vi "Read Config Unitest.vi"(8 "error in (no error)":errorcluster, 11 "main ref":T1) -> (0 "error out":errorcluster)   [LabVIEW 2025]
uses:
  controls/LAB-IQ UI Data.ctl
  Config file  FGV Unitest enum.ctl
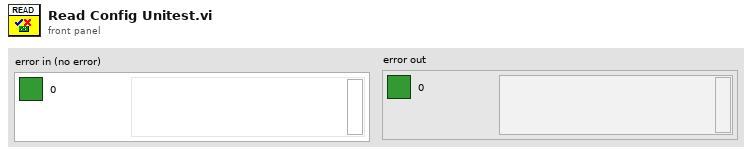
[diagram p1: front panel]
types:
  T1 = typedef "LAB-IQ UI Data.ctl" = cluster{"Main Home Screen":cluster{"GUI":refnum<vi>, "Platform Settings":refnum<vi>, "Configure":refnum<vi>, "Home":refnum<vi>, "EXIT":refnum<vi>, "service 2":refnum<vi>, "MainPage":refnum<vi>, "Analysis":refnum<vi>}, "Platform Settings":cluster{"mm/s  Surge":refnum<vi>, "Update Surge Speed":refnum<vi>, "Drive Error":refnum<vi>, "Disable Axis Jog Soft Limits":refnum<vi>, "mm/s  Sway":refnum<vi>, "Sway and Surge COM Status":refnum<vi>, "Heave COM Status":refnum<vi>, "Enable Platform":refnum<vi>, "Surge Forward Main":refnum<vi>, "Sway Right Main":refnum<vi>, "Sway Left Main":refnum<vi>, "Heave Down Main":refnum<vi>, "Heave Up main":refnum<vi>, "Update Sway Speed":refnum<vi>, "Update Heave Speed":refnum<vi>, "mm/s Heave":refnum<vi>, "mm/sec":refnum<vi>, "mm":refnum<vi>, "Surge Backward Main":refnum<vi>}, "Analysis Screen":cluster{"Analysis Home":refnum<vi>, "Surface Analysis":refnum<vi>, "Imaging":refnum<vi>, "Image Analysis":refnum<vi>, "Post Analysis":refnum<vi>}, "Config Screen":cluster{"Select Load Head":refnum<vi>, "Notes :":refnum<vi>, "FILE":refnum<vi>, "Sample ID :":refnum<vi>, "Operator ID :":refnum<vi>, "Operator Name :":refnum<vi>, "Auto":refnum<vi>}, "Motion Module":cluster{"zNL":refnum<vi>, "NL disp":refnum<vi>, "Rotary Tab":refnum<vi>, "Motion Direction:  3":refnum<vi>, "E.Velocity 2":refnum<vi>, "e.v/ssr 2":refnum<vi>, "Enter Fixed E.Velocity 2":refnum<vi>, "Enter Final SRR 2":refnum<vi>, "Enter initial SRR 2":refnum<vi>, "Enter Fixed SRR 2":refnum<vi>, "Enter the Final E.Velocity (m/s) 2":refnum<vi>, "Enter initial E.Velocity (m/s) 2":refnum<vi>, "Final Speed (RPM) 3":refnum<vi>, "Initial Speed (RPM) 2":refnum<vi>, "Enter the Final Velocity (m/s) 3":refnum<vi>, "Enter initial Velocity (m/s)  3":refnum<vi>, "Ramp Up 2":refnum<vi>, "TEST SELECTION":refnum<vi>, "SPEED SELECTION : ":refnum<vi>, "Angular Oscillation Set":refnum<vi>, "Traction":refnum<vi>, "Step Speed":refnum<vi>, "StepTable For Load-Speed":refnum<vi>, "StepTable For Speed":refnum<vi>, "Surge Forward MM":refnum<vi>, "Surge Backward MM":refnum<vi>, "M3 Image":refnum<vi>, "String 39":refnum<vi>, "Sway Left MM":refnum<vi>, "Sway Right MM":refnum<vi>, "Disable Axis Jog Soft Limits":refnum<vi>, "mm":refnum<vi>, "Heave Down MM":refnum<vi>, "Heave Up MM":refnum<vi>, "Wear Track Diameter (mm)":refnum<vi>, "Set WTD":refnum<vi>, "HomeScratch":refnum<vi>, "HomeRot":refnum<vi>, "PlaceModule":refnum<vi>, "Enter the Angle (Deg)":refnum<vi>, "Enter the Frequency (Hz)":refnum<vi>, "Motion Mode:":refnum<vi>, "LR Sway":refnum<vi>, "Rot Hor":refnum<vi>, "Scratch":refnum<vi>, "LR Cam":refnum<vi>, "MMBack":refnum<vi>, "MMNext":refnum<vi>, "Rot Ver":refnum<vi>, "Rotary Module Selection":refnum<vi>, "calculate rotary":refnum<vi>, "SPEED SELECTION : rotary":refnum<vi>, "Import 2":refnum<vi>, "Save 2":refnum<vi>, "File Path :  2":refnum<vi>, "String 45":refnum<vi>, "StepTable For Speed 3":refnum<vi>, "Enter the Speed(mm/sec)":refnum<vi>, "Enter the Speed(RPM)":refnum<vi>, "Enter Scratch Speed (mm/s):":refnum<vi>, "SwaySpeed Set":refnum<vi>, "Scartch Offset":refnum<vi>, "Motion type:":refnum<vi>, "HomeScratch 2":refnum<vi>, "Enter Scratch length (mm):":refnum<vi>, "Wear Track Diameter":refnum<vi>, "Rotary Speed Exced":refnum<vi>, "Scratch Mode":refnum<vi>, "No of Scratch":refnum<vi>}, "Environmental control":cluster{"Humidity  Status  3":refnum<vi>, "Low Temp  Status  2":refnum<vi>, "TK4 status 2":refnum<vi>, "Stage Temperature":refnum<vi>, "Sample Temperature":refnum<vi>, "Humidity (Amb)":refnum<vi>, "Clear List":refnum<vi>, "Add to list":refnum<vi>, "Wear":refnum<vi>, "Vibration":refnum<vi>, "Humidity (Chamber)":refnum<vi>, "Temperature (Chamber)":refnum<vi>, "ECR ":refnum<vi>, "Temperature (Amb)":refnum<vi>, "Microphone":refnum<vi>, "Acoustic Emission 3":refnum<vi>, "SNext":refnum<vi>, "APBack":refnum<vi>, "Enter the Temperature (°C):":refnum<vi>, "Enter the Stage \nTemperature (°C):":refnum<vi>, "Enter the Humidity (%Rh):":refnum<vi>, "Low Temp":refnum<vi>, "High Temp":refnum<vi>, "Humidity":refnum<vi>, "Sensors Picked":refnum<vi>}, "About Screen":cluster{"Password":refnum<vi>, "Home Service":refnum<vi>, "Advanced Setting":refnum<vi>, "About Tab":refnum<vi>, "ECR Port:":refnum<vi>, "Ramp Port:":refnum<vi>, "Installation/Replacement completed":refnum<vi>, "Loahead":refnum<vi>, "Heave and Surge COM Port:":refnum<vi>, "Sway COM Port:":refnum<vi>, "Temp Modbus:":refnum<vi>, "Humidity Port:":refnum<vi>, "Edit Gain Constants":refnum<vi>, "Save Gain Constants":refnum<vi>}, "Main Screen":cluster{"Main Screen Tab":refnum<vi>, "Angle and Frequency":refnum<vi>, "Stroke (mm)":refnum<vi>, "Angle (Deg)":refnum<vi>, "Main Speed Tab":refnum<vi>, "MTM MOTOR DISPLAY":refnum<vi>, "Disc Speed (m/sec)":refnum<vi>, "Ball Speed (m/sec)":refnum<vi>, "Disc Speed (RPM)":refnum<vi>, "Ball Speed (RPM)":refnum<vi>, "SPEED TAB":refnum<vi>, "Speed (m/sec)":refnum<vi>, "Set Speed (m/sec)":refnum<vi>, "Speed (RPM)":refnum<vi>, "Set Speed":refnum<vi>, "Time Tab":refnum<vi>, "Time ( HH:MM:SS ) 2":refnum<vi>, "Test Duration":refnum<vi>, "Test Duration 4":refnum<vi>, "TEST CYCLE":refnum<vi>, "TOTAL CYCLES":refnum<vi>, "Set Load (N)":refnum<vi>, "Temp Tabs":refnum<vi>, "Heater":refnum<vi>, "TK4 status":refnum<vi>, "ChamberTemp":refnum<vi>, "SetTmp":refnum<vi>, "Controller  Status":refnum<vi>, "ChamberTemp 2":refnum<vi>, "SetTmp 2":refnum<vi>, "Controller  Status 2":refnum<vi>, "ChamberTemp 3":refnum<vi>, "SetTmp 3":refnum<vi>, "Cooling":refnum<vi>, "Load Communication":refnum<vi>, "Ambient \nTemperature":refnum<vi>, "HumCOMStatus":refnum<vi>, "Ambient\n Humidity":refnum<vi>, "Freq (Hz)":refnum<vi>, "Load En":refnum<vi>, "NLt":refnum<vi>, "zNL 2":refnum<vi>, "Humidity On":refnum<vi>, "humidity disp":refnum<vi>, "Set Humidity":refnum<vi>, "NL disp 2":refnum<vi>, "Humidity On 2":refnum<vi>, "humidity disp 2":refnum<vi>, "Set Humidity 2":refnum<vi>, "NL disp 3":refnum<vi>, "AppLoadSeq scratch":refnum<vi>, "Stop Scratch":refnum<vi>, "ClrLog":refnum<vi>, "Trip Log":refnum<vi>, "STOP":refnum<vi>, "Start Test":refnum<vi>, "Test status":refnum<vi>, "AR Led":refnum<vi>, "Data":refnum<vi>, "Health":refnum<vi>, "Sway COM Status":refnum<vi>, "Heave COM Status":refnum<vi>, "Grp Tab":refnum<vi>, "Sub Graph":refnum<vi>, "SD (mm)":refnum<vi>, "Siliding distance Reset Graph":refnum<vi>, "SDGp":refnum<vi>, "Humidity Reset Graph":refnum<vi>, "HumrGp":refnum<vi>, "Acoustic Emission (mV)":refnum<vi>, "Aqucostic Reset Graph":refnum<vi>, "gACQUOS":refnum<vi>, "ECR RESET":refnum<vi>, "ECR":refnum<vi>, "Temperature Reset":refnum<vi>, "Acoustic Emission (mV) 2":refnum<vi>, "Aqucostic Reset Graph 2":refnum<vi>, "gACQUOS 2":refnum<vi>, "ECR RESET 2":refnum<vi>, "ECR 2":refnum<vi>, "Temperature Reset 2":refnum<vi>, "Temperature (deg c)":refnum<vi>, "Speed Reset Graph":refnum<vi>, "Speed Tab":refnum<vi>, "MTM DISC  SPEED":refnum<vi>, "MTM BALL SPEED":refnum<vi>, "speed mm/sec":refnum<vi>, "Hymidity":refnum<vi>, "Humidity Disable trip":refnum<vi>, "CoF Trip  2":refnum<vi>, "Depth Trip":refnum<vi>, "Weart Deapth":refnum<vi>, "Depth Reset Graph":refnum<vi>, "Weart":refnum<vi>, "Depthz":refnum<vi>, "Depth (µm)":refnum<vi>, "WearGp":refnum<vi>, "NL Trip 2":refnum<vi>, "Load pid":refnum<vi>, "Load Disable Trip":refnum<vi>, "Load Reset Graph":refnum<vi>, "NL Display 4":refnum<vi>, "Main Chart 3":refnum<vi>, "BACK":refnum<vi>, "Depth Trip 2":refnum<vi>, "COF TRIP ":refnum<vi>, "Friction Force (N)":refnum<vi>, "FF Reset Graph":refnum<vi>, "FF Disable Trip":refnum<vi>, "FF TRIP":refnum<vi>, "COF Disable Trip":refnum<vi>, "COF Reset Graph":refnum<vi>, "Start Test Temp":refnum<vi>, "zFF":refnum<vi>, "Friction Force (N) Graph":refnum<vi>, "Coefficient of Friction":refnum<vi>, "Scratch Start Test":refnum<vi>, "FF Tab":refnum<vi>, "Cyclic Friction Force (N)":refnum<vi>, "CZ FF":refnum<vi>, "Cyclic Friction Force (N) Graph":refnum<vi>, "Cyclic Coefficient of Friction":refnum<vi>, "Cyclic FF TRIP":refnum<vi>, "Cyclic FF Disable Trip":refnum<vi>, "cyclic COF Disable Trip":refnum<vi>, "cyclic COF TRIP":refnum<vi>, "cyclic COF Reset Graph":refnum<vi>, "Cyclic FF Reset Graph":refnum<vi>, "Test Trip":refnum<vi>, "Multi Scratch Pass":refnum<vi>, "Scratch Start Recording":refnum<vi>}, "Loading":cluster{"Indentation":refnum<vi>, "Reference Sample":refnum<vi>, "Load Cell Communication Slide":refnum<vi>, "com 3":refnum<vi>, "com":refnum<vi>, "DecaForce COM Status":refnum<vi>, "Update":refnum<vi>, "Clear 3":refnum<vi>, "seq":refnum<vi>, "Stribeck table":refnum<vi>, "Stribeck Table  For loading":refnum<vi>, "Loading Mode":refnum<vi>, "Enter the Final Load (N)":refnum<vi>, "Enter the CoF Trip":refnum<vi>, "Enter the Friction Force Trip":refnum<vi>, "Enter the Normal load Trip":refnum<vi>, "Enter the Load  (N)":refnum<vi>, "KiloForce":refnum<vi>, "DecaForce ":refnum<vi>, "MicroForce":refnum<vi>, "LHBack":refnum<vi>, "LHNext":refnum<vi>, "Enter the Loading Rate (N/min)":refnum<vi>, "Message":refnum<vi>, "Warning 2":refnum<vi>, "SSP 0.75":refnum<vi>, "SSP 0.5":refnum<vi>, "SSP 0.3":refnum<vi>, "Warning":refnum<vi>, "gui GIF":refnum<vi>, "Communication is established":refnum<vi>, "AppLoad 4":refnum<vi>, "Multipoint":refnum<vi>, "Load Selection":refnum<vi>}, "PID":cluster{"Ramp MulFac":refnum<vi>, "pulses LoadDiffRamp(2..10)":refnum<vi>, "PulseControlRamp(diff<=3N)":refnum<vi>, "SetLoadDeadband(%) Load(0-10N)":refnum<vi>, "PID gains out delay (microForce)":refnum<vi>, "Ramp":refnum<vi>, "Gain 2":refnum<vi>, "pulses LoadDiff(2..10)":refnum<vi>, "pulses LoadDiff(11..50)":refnum<vi>, "PulseControl(diff<=3N)":refnum<vi>, "SetLoadDeadband(%)  2":refnum<vi>, "Dummy Run":refnum<vi>, "Vertical load (N)":refnum<vi>, "AutoTune":refnum<vi>, "Offset 3 ":refnum<vi>, "apply load":refnum<vi>, "Offset  3":refnum<vi>, "apply load 2":refnum<vi>, "Enter ByPass Load":refnum<vi>, "reinit 3":refnum<vi>, "output range delay":refnum<vi>, "PID gains out delay":refnum<vi>, "Bypass Load":refnum<vi>, "pulsesSent":refnum<vi>, "pulses ":refnum<vi>, "actpid":refnum<vi>, "gFF Rot":refnum<vi>, "pulses LoadDiff(21..1000)":refnum<vi>, "Delay":refnum<vi>, "deadband":refnum<vi>}, "Config Parameters":cluster{"Tab Control 3":refnum<vi>, "Tab Control 19":refnum<vi>, "SAMPLES":refnum<vi>, "Re-initilaize":refnum<vi>, "Filter ON/OFF":refnum<vi>, "TracHomeSurgeOffsetCounts 10MM":refnum<vi>, "TracHomeSwayOffsetCounts 10MM":refnum<vi>, "Acoustic Emission:":refnum<vi>, "Apply Filter (FF)":refnum<vi>, "Filter% 2":refnum<vi>, "Apply Filter (Load)":refnum<vi>, "Filter% ":refnum<vi>, "Sway distance (mm)":refnum<vi>, "Surge distance (mm)":refnum<vi>, "DataSavingLoopDelay(ms)":refnum<vi>, "SAVE 2":refnum<vi>, "Enter Distance":refnum<vi>, "Sway Counts:":refnum<vi>, "Distance (mm): 3":refnum<vi>, "Surge Counts:":refnum<vi>, "Distance (mm): 2":refnum<vi>, "Distance (mm):":refnum<vi>, "Heave Counts:":refnum<vi>, "LRMHomeSurgeOffsetCounts":refnum<vi>, "LRMHomeSwayOffsetCounts":refnum<vi>, "TracHomeSurgeOffsetCounts 20MM":refnum<vi>, "TracHomeSwayOffsetCounts 20MM":refnum<vi>, "RotHomeSwayOffsetCounts":refnum<vi>, "RotHomeSurgeOffsetCounts":refnum<vi>, "Heave distance":refnum<vi>, "Zmm":refnum<vi>, "Heave Pulses/mm":refnum<vi>, "Surge Pulses/mm":refnum<vi>, "Sway Pulses/mm":refnum<vi>, "Heave Pitch":refnum<vi>, "Surge Pitch":refnum<vi>, "Sway Pitch":refnum<vi>, "Heave PPR":refnum<vi>, "Surge PPR":refnum<vi>, "Sway PPR":refnum<vi>, "Tab Control 5":refnum<vi>, "Tab Control 14":refnum<vi>, "Tab Control 26":refnum<vi>, "AE":refnum<vi>, "Heave Loop Delay":refnum<vi>, "Heave PID Speed":refnum<vi>, "Surge Jog Speed":refnum<vi>, "Heave Jog Speed":refnum<vi>, "Sway Loop Delay":refnum<vi>, "Sway PID Speed":refnum<vi>, "Sway Jog Speed":refnum<vi>, "DEPTH TRIP VALUE":refnum<vi>, "LOAD TRIP VALUE":refnum<vi>, "DEPTH TRIP   ENABLE":refnum<vi>, "LOAD TRIP  ENABLE":refnum<vi>, "CYCLIC FF TRIP VALUE":refnum<vi>, "FF TRIP VALUE":refnum<vi>, "CYCLIC CoF TRIP VALUE":refnum<vi>, "COF TRIP VALUE":refnum<vi>, "CYCLIC COF TRIP  ENABLE":refnum<vi>, "CYCLIC FF TRIP  ENABLE":refnum<vi>, "FF TRIP  ENABLE":refnum<vi>, "COF TRIP  ENABLE":refnum<vi>}, "Loading Com Port":cluster{"ClearAll":refnum<vi>, "Mz(Nm)":refnum<vi>, "My(Nm)":refnum<vi>, "Mx(Nm)":refnum<vi>, "Save Dwell":refnum<vi>, "Mx ":refnum<vi>, "My ":refnum<vi>, "Mz":refnum<vi>, "Fx(N)":refnum<vi>, "Fy(N)":refnum<vi>, "Fz(N)":refnum<vi>, "ZeroAll":refnum<vi>, "Acq Delay (ms)":refnum<vi>, "Burst Delay (ms)":refnum<vi>, "model":refnum<vi>, "SN":refnum<vi>, "FFx(N)":refnum<vi>, "Sensor IP":refnum<vi>, "Port":refnum<vi>, "FFy(N)":refnum<vi>, "Load(N)":refnum<vi>, "delete Handle":refnum<vi>, "Create Handle":refnum<vi>, "ft_data":refnum<vi>, "ft_range":refnum<vi>, "ft_data 2":refnum<vi>, "stop 6":refnum<vi>, "running_flag":refnum<vi>, "ft_udp_handle":refnum<vi>, "get-data-return":refnum<vi>, "get-range-return":refnum<vi>, "zero-return":refnum<vi>, "filter-return":refnum<vi>, "initial-return":refnum<vi>, "deleteHandle-result":refnum<vi>, "Load Cell Temp":refnum<vi>}, "Heave AND Surge":cluster{"SURGE POSE":refnum<vi>, "error out Read":refnum<vi>, "HEAVE POSE":refnum<vi>, "State":refnum<vi>, "Homed":refnum<vi>, "Sequence ID":refnum<vi>, "error out Write":refnum<vi>, "faultCode":refnum<vi>, "Ack ID":refnum<vi>, "SPEED":refnum<vi>, "Distance":refnum<vi>, "Mode Command":refnum<vi>, "Heave and Surge Read":refnum<vi>, "Read Heave Temp":refnum<vi>, "Spare 15":refnum<vi>, "Spare 14":refnum<vi>, "Spare 13":refnum<vi>, "Spare 12":refnum<vi>, "Spare 11":refnum<vi>, "Spare 10":refnum<vi>, "Spare 9":refnum<vi>, "Spare 8":refnum<vi>, "Spare 7":refnum<vi>, "Spare 6":refnum<vi>, "Spare 5":refnum<vi>, "Spare 4":refnum<vi>, "Spare 2":refnum<vi>, "Spare 1":refnum<vi>, "Node Id":refnum<vi>, "Spare 3":refnum<vi>, "SPARE 4":refnum<vi>, "SPARE 3":refnum<vi>, "SPARE 2":refnum<vi>, "SPARE 1":refnum<vi>, "fwMajor":refnum<vi>, "fwMinor":refnum<vi>, "Manual Write":refnum<vi>, "Heave and Surge Write":refnum<vi>}, "New PID LOGIC":cluster{"Fine Tune Zone":refnum<vi>, "PID SDelay":refnum<vi>, "Max_pos_limit":refnum<vi>, "Min_pos_limit":refnum<vi>, "i_limit":refnum<vi>, "pct_scale":refnum<vi>, "Deadband":refnum<vi>, "Kd":refnum<vi>, "Ki":refnum<vi>, "Kp":refnum<vi>, "Current Position":refnum<vi>, "Set Load":refnum<vi>, "Current Load":refnum<vi>, "Pulse delta":refnum<vi>, "Init Step":refnum<vi>, "Max Step Linit":refnum<vi>}, "SWAY ":cluster{"fwMajor":refnum<vi>, "Homed":refnum<vi>, "Rotary POSE":refnum<vi>, "State":refnum<vi>, "SWAY POSE":refnum<vi>, "Ack ID":refnum<vi>, "faultCode":refnum<vi>, "Node Id":refnum<vi>, "fwMinor":refnum<vi>, "Spare 6":refnum<vi>, "Spare 5":refnum<vi>, "Spare 4":refnum<vi>, "Spare 3":refnum<vi>, "Spare 2":refnum<vi>, "Spare 1":refnum<vi>, "Spare 7":refnum<vi>, "SPARE  5":refnum<vi>, "error out Write  SWAY ":refnum<vi>, "error out Read SWAY ":refnum<vi>, "Manual Write SWAY ":refnum<vi>, "SWAY WRITE":refnum<vi>, "SPARE  4":refnum<vi>, "SPARE  3":refnum<vi>, "SPARE 2":refnum<vi>, "SPARE 1":refnum<vi>, "Spare 15":refnum<vi>, "Spare 14":refnum<vi>, "Spare 13":refnum<vi>, "Spare 12":refnum<vi>, "Spare 11":refnum<vi>, "Spare 9":refnum<vi>, "Spare 8":refnum<vi>, "SPEED":refnum<vi>, "Distance":refnum<vi>, "Mode Command":refnum<vi>, "Sequence ID":refnum<vi>, "SWAY READ":refnum<vi>, "Spare 10":refnum<vi>, "Read SWAY Temp":refnum<vi>}, "Analysis Screen":cluster{"Analysis Home":refnum<vi>, "Refresh 2":refnum<vi>, "MEAN 4":refnum<vi>, "SD 4":refnum<vi>, "VARIANCE 4":refnum<vi>, "MEAN  3":refnum<vi>, "SD  3":refnum<vi>, "VARIANCE  3":refnum<vi>, "MEAN 2":refnum<vi>, "SD  2":refnum<vi>, "VARIANCE 2":refnum<vi>, "MEAN":refnum<vi>, "SD":refnum<vi>, "VARIANCE":refnum<vi>, "File 4 Discription":refnum<vi>, "OPEN 4":refnum<vi>, "File Name 4":refnum<vi>, "OPEN 3":refnum<vi>, "File 3 Discription":refnum<vi>, "File Name 3":refnum<vi>, "Y-AXIS":refnum<vi>, "X-AXIS":refnum<vi>, "XY Graph":refnum<vi>, "File Name 2":refnum<vi>, "File Name 1":refnum<vi>, "OPEN 2":refnum<vi>, "OPEN 1":refnum<vi>, "File 1 Discription ":refnum<vi>, "File 2 Discription":refnum<vi>, "Export":refnum<vi>, "File Format":refnum<vi>}}
  T2 = typedef "Config file  FGV Unitest enum.ctl" = enum16{"OPEN", "READ", "WRITE", "CLOSE"}
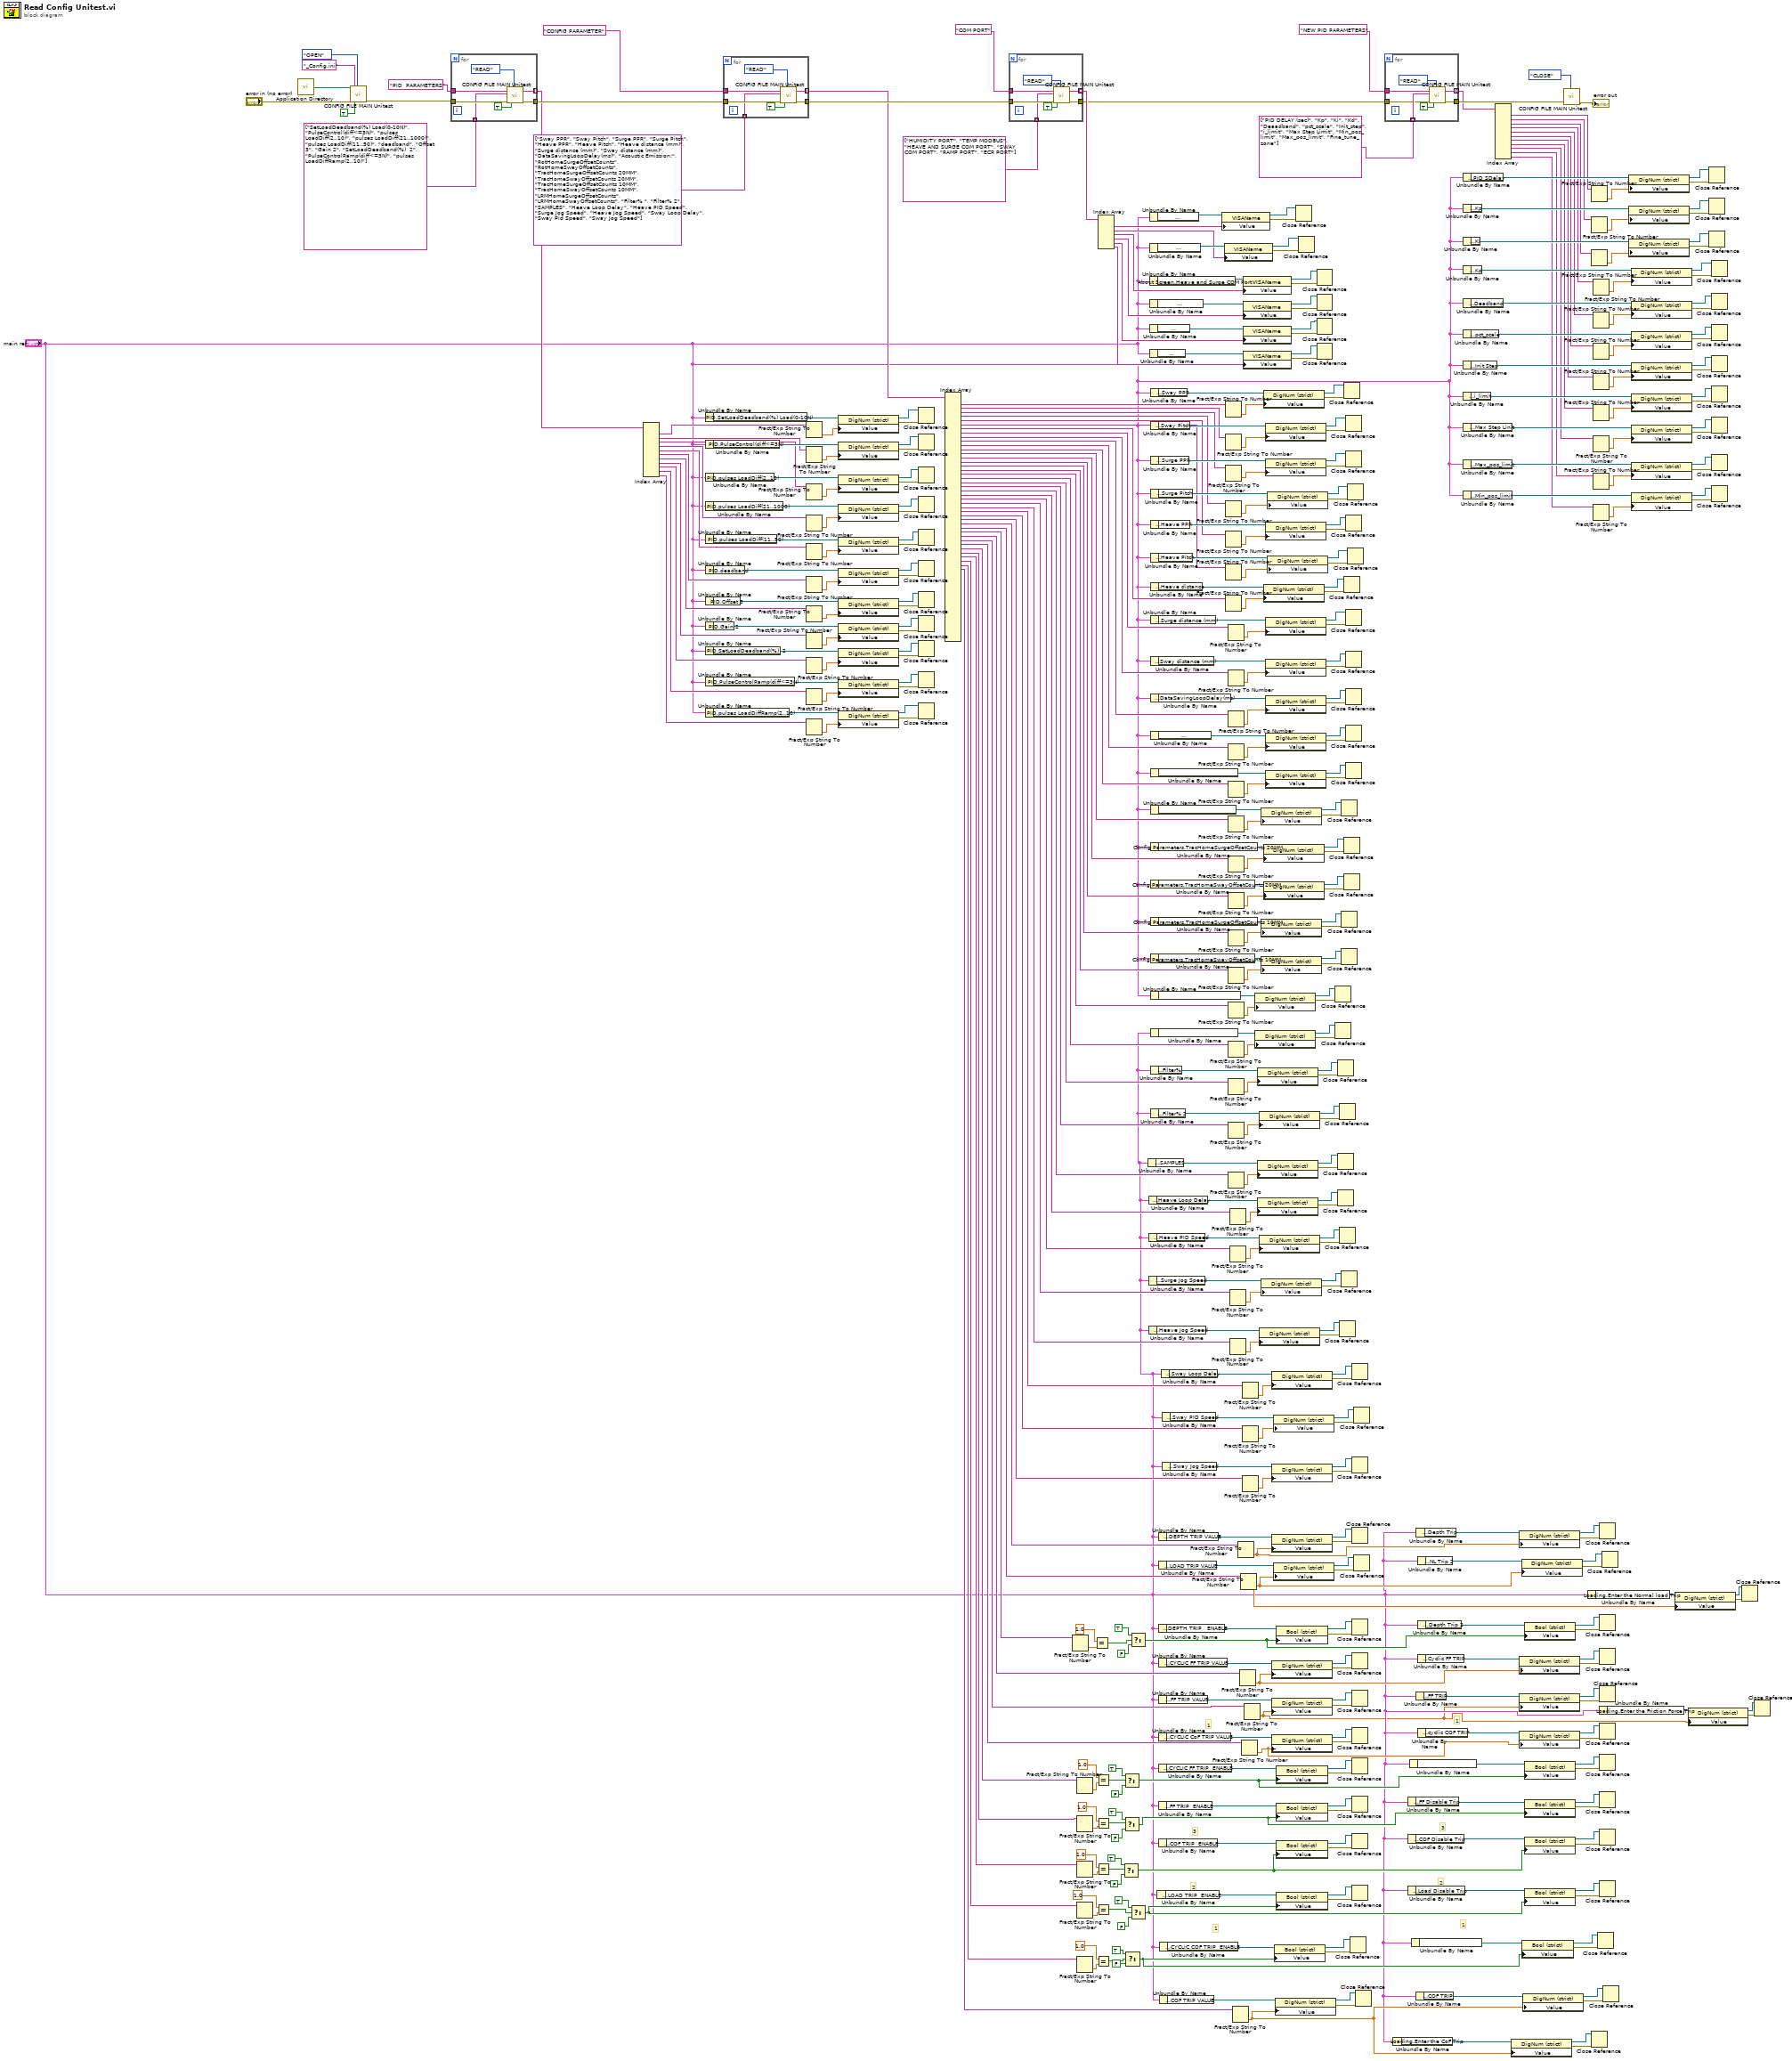
[diagram p0: block diagram]
diagram:
  # "3"
  # "2"
  # "1"
  # "1"
  # "3"
  # "2"
  # "1"
  # "1"
  n1 = call <vilib>:"Application Directory.vi"() -> ("Application Directory"=w435:path)
  n2 = call "CONFIG FILE MAIN Unitest.vi"("File Path"=w435, "error in"="error in (no error)", "file name"="_Config.ini", "PARAMETER/CONFIG"=TRUE, "Config Enum"=Config_file__FGV_Unitest_enum."OPEN") -> ("error out"=w434:errorcluster)  [unwired: 13 in, 1 out]
  n3 = for {
    tunnel: w434 -> [w446]
    tunnel: "PID  PARAMETERS" ("WRITE /READ SECTION") -> [w445]
    tunnel: string[] ["SetLoadDeadband(%) Load(0-10N)", "PulseControl(diff<=3N)", "pulses LoadDiff(2..10)", "pulses LoadDiff(21..1000)", "pulses LoadDiff(11..50)", "deadband", "Offset  3", "Gain 2", "SetLoadDeadband(%)  2", "PulseControlRamp(diff<=3N)", "pulses LoadDiffRamp(2..10)"] -> [w441] mode=indexing
    tunnel: [w444] -> w431
    tunnel: [w440] -> w244 mode=indexing
    n4 = call "CONFIG FILE MAIN Unitest.vi"("WRITE /READ SECTION"=w445, "READ KEY"=w441, "error in"=w446, "PARAMETER/CONFIG"=TRUE, "Config Enum"=Config_file__FGV_Unitest_enum."READ") -> ("READ VALUE"=w440:string, "error out"=w444:errorcluster)  [unwired: 13 in]
  }
  n5 = Index Array(array=w244) -> (element #1=w243:string, element #2=w242:string, element #3=w241:string, element #4=w240:string, element #5=w239:string, element #6=w238:string, element #7=w237:string, element #8=w236:string, element #9=w235:string, element #10=w234:string, element #11=w233:string)  [unwired: 11 in]
  n6 = Unbundle By Name("main ref") -> ("PID.SetLoadDeadband(%) Load(0-10N)"=w425:refnum<vi>)
  n7 = Unbundle By Name("main ref") -> ("PID.PulseControl(diff<=3N)"=w420:refnum<vi>)
  n8 = Unbundle By Name("main ref") -> ("PID.pulses LoadDiff(2..10)"=w419:refnum<vi>)
  n9 = Unbundle By Name("main ref") -> ("PID.pulses LoadDiff(21..1000)"=w414:refnum<vi>)
  n10 = Unbundle By Name("main ref") -> ("PID.pulses LoadDiff(11..50)"=w413:refnum<vi>)
  n11 = Unbundle By Name("main ref") -> ("PID.deadband"=w408:refnum<vi>)
  n12 = Unbundle By Name("main ref") -> ("PID.Offset 3"=w407:refnum<vi>)
  n13 = Unbundle By Name("main ref") -> ("PID.Gain 2"=w402:refnum<vi>)
  n14 = Unbundle By Name("main ref") -> ("PID.SetLoadDeadband(%)  2"=w401:refnum<vi>)
  n15 = Unbundle By Name("main ref") -> ("PID.PulseControlRamp(diff<=3N)"=w397:refnum<vi>)
  n16 = Unbundle By Name("main ref") -> ("PID.pulses LoadDiffRamp(2..10)"=w395:refnum<vi>)
  n17 = for {
    tunnel: w431 -> [w453]
    tunnel: "CONFIG PARAMETER" ("WRITE /READ SECTION") -> [w452]
    tunnel: [w451] -> w429
    tunnel: string[] ["Sway PPR", "Sway Pitch", "Surge PPR", "Surge Pitch", "Heave PPR", "Heave Pitch", "Heave distance (mm)", "Surge distance (mm)", "Sway distance (mm)", "DataSavingLoopDelay(ms)", "Acoustic Emission:", "RotHomeSurgeOffsetCounts", "RotHomeSwayOffsetCounts", "TracHomeSurgeOffsetCounts 20MM", "TracHomeSwayOffsetCounts 20MM", "TracHomeSurgeOffsetCounts 10MM", "TracHomeSwayOffsetCounts 10MM", "LRMHomeSurgeOffsetCounts", "LRMHomeSwayOffsetCounts", "Filter% ", "Filter% 2", "SAMPLES", "Heave Loop Delay", "Heave PID Speed", "Surge Jog Speed", "Heave Jog Speed", "Sway Loop Delay", "Sway Pid Speed", "Sway Jog Speed"] -> [w448] mode=indexing
    tunnel: [w447] -> w300 mode=indexing
    n18 = call "CONFIG FILE MAIN Unitest.vi"("WRITE /READ SECTION"=w452, "READ KEY"=w448, "error in"=w453, "PARAMETER/CONFIG"=TRUE, "Config Enum"=Config_file__FGV_Unitest_enum."READ") -> ("READ VALUE"=w447:string, "error out"=w451:errorcluster)  [unwired: 13 in]
  }
  n19 = Fract/Exp String To Number(string=w243) -> (number=w255:dbl)  [unwired: 3 in, 1 out]
  n20 = Fract/Exp String To Number(string=w242) -> (number=w254:dbl)  [unwired: 3 in, 1 out]
  n21 = Fract/Exp String To Number(string=w241) -> (number=w253:dbl)  [unwired: 3 in, 1 out]
  n22 = Fract/Exp String To Number(string=w240) -> (number=w252:dbl)  [unwired: 3 in, 1 out]
  n23 = Fract/Exp String To Number(string=w239) -> (number=w251:dbl)  [unwired: 3 in, 1 out]
  n24 = Fract/Exp String To Number(string=w238) -> (number=w250:dbl)  [unwired: 3 in, 1 out]
  n25 = Fract/Exp String To Number(string=w237) -> (number=w249:dbl)  [unwired: 3 in, 1 out]
  n26 = Fract/Exp String To Number(string=w236) -> (number=w248:dbl)  [unwired: 3 in, 1 out]
  n27 = Fract/Exp String To Number(string=w235) -> (number=w247:dbl)  [unwired: 3 in, 1 out]
  n28 = Fract/Exp String To Number(string=w234) -> (number=w246:dbl)  [unwired: 3 in, 1 out]
  n29 = Fract/Exp String To Number(string=w233) -> (number=w245:dbl)  [unwired: 3 in, 1 out]
  n30 = property class="DigNum (strict)"(reference=w425, "Value"=w255) -> (reference out=w423:refnum<vi>, error out=w424:errorcluster)  [unwired: 1 in]
  n31 = property class="DigNum (strict)"(reference=w420, "Value"=w254) -> (reference out=w422:refnum<vi>, error out=w421:errorcluster)  [unwired: 1 in]
  n32 = property class="DigNum (strict)"(reference=w419, "Value"=w253) -> (reference out=w417:refnum<vi>, error out=w418:errorcluster)  [unwired: 1 in]
  n33 = property class="DigNum (strict)"(reference=w414, "Value"=w252) -> (reference out=w416:refnum<vi>, error out=w415:errorcluster)  [unwired: 1 in]
  n34 = property class="DigNum (strict)"(reference=w413, "Value"=w251) -> (reference out=w411:refnum<vi>, error out=w412:errorcluster)  [unwired: 1 in]
  n35 = property class="DigNum (strict)"(reference=w408, "Value"=w250) -> (reference out=w410:refnum<vi>, error out=w409:errorcluster)  [unwired: 1 in]
  n36 = property class="DigNum (strict)"(reference=w407, "Value"=w249) -> (reference out=w405:refnum<vi>, error out=w406:errorcluster)  [unwired: 1 in]
  n37 = property class="DigNum (strict)"(reference=w402, "Value"=w248) -> (reference out=w404:refnum<vi>, error out=w403:errorcluster)  [unwired: 1 in]
  n38 = property class="DigNum (strict)"(reference=w401, "Value"=w247) -> (reference out=w399:refnum<vi>, error out=w400:errorcluster)  [unwired: 1 in]
  n39 = property class="DigNum (strict)"(reference=w397, "Value"=w246) -> (reference out=w396:refnum<vi>, error out=w398:errorcluster)  [unwired: 1 in]
  n40 = property class="DigNum (strict)"(reference=w395, "Value"=w245) -> (reference out=w393:refnum<vi>, error out=w394:errorcluster)  [unwired: 1 in]
  n41 = Close Reference(reference=w423, error in (no error)=w424) -> ()  [unwired: 1 out]
  n42 = Close Reference(reference=w422, error in (no error)=w421) -> ()  [unwired: 1 out]
  n43 = Close Reference(reference=w417, error in (no error)=w418) -> ()  [unwired: 1 out]
  n44 = Close Reference(reference=w416, error in (no error)=w415) -> ()  [unwired: 1 out]
  n45 = Close Reference(reference=w411, error in (no error)=w412) -> ()  [unwired: 1 out]
  n46 = Close Reference(reference=w410, error in (no error)=w409) -> ()  [unwired: 1 out]
  n47 = Close Reference(reference=w405, error in (no error)=w406) -> ()  [unwired: 1 out]
  n48 = Close Reference(reference=w404, error in (no error)=w403) -> ()  [unwired: 1 out]
  n49 = Close Reference(reference=w399, error in (no error)=w400) -> ()  [unwired: 1 out]
  n50 = Close Reference(reference=w396, error in (no error)=w398) -> ()  [unwired: 1 out]
  n51 = Close Reference(reference=w393, error in (no error)=w394) -> ()  [unwired: 1 out]
  n52 = Index Array(array=w300) -> (element #1=w299:string, element #2=w298:string, element #3=w297:string, element #4=w296:string, element #5=w295:string, element #6=w294:string, element #7=w293:string, element #8=w292:string, element #9=w291:string, element #10=w290:string, element #11=w289:string, element #12=w288:string, element #13=w287:string, element #14=w286:string, element #15=w285:string, element #16=w284:string, element #17=w283:string, element #18=w282:string, element #19=w281:string, element #20=w280:string, element #21=w279:string, element #22=w278:string, element #23=w216:string, element #24=w215:string, element #25=w214:string, element #26=w213:string, element #27=w139:string, element #28=w138:string, element #29=w137:string, element #30=w87:string, element #31=w86:string, element #32=w85:string, element #33=w84:string, element #34=w83:string, element #35=w82:string, element #36=w81:string, element #37=w80:string, element #38=w79:string, element #39=w78:string, element #40=w77:string, element #41=w23:string)  [unwired: 58 in, 17 out]
  n53 = for {
    tunnel: w429 -> [w460]
    tunnel: "COM PORT" ("WRITE /READ SECTION") -> [w459]
    tunnel: [w458] -> w211
    tunnel: string[] ["HUMIDITY PORT", "TEMP MODBUS", "HEAVE AND SURGE COM PORT", "SWAY COM PORT", "RAMP PORT", "ECR PORT"] -> [w455] mode=indexing
    tunnel: [w454] -> w307 mode=indexing
    n54 = call "CONFIG FILE MAIN Unitest.vi"("WRITE /READ SECTION"=w459, "READ KEY"=w455, "error in"=w460, "PARAMETER/CONFIG"=TRUE, "Config Enum"=Config_file__FGV_Unitest_enum."READ") -> ("READ VALUE"=w454:string, "error out"=w458:errorcluster)  [unwired: 13 in]
  }
  n55 = Fract/Exp String To Number(string=w85) -> (number=w99:dbl)  [unwired: 3 in, 1 out]
  n56 = Fract/Exp String To Number(string=w81) -> (number=w100:dbl)  [unwired: 3 in, 1 out]
  n57 = Fract/Exp String To Number(string=w80) -> (number=w98:dbl)  [unwired: 3 in, 1 out]
  n58 = Fract/Exp String To Number(string=w79) -> (number=w97:dbl)  [unwired: 3 in, 1 out]
  n59 = Fract/Exp String To Number(string=w78) -> (number=w96:dbl)  [unwired: 3 in, 1 out]
  n60 = Fract/Exp String To Number(string=w77) -> (number=w95:dbl)  [unwired: 3 in, 1 out]
  n61 = Equal?(x=1.0, y=w99) -> (x = y?=w60:bool)
  n62 = Equal?(x=1.0, y=w100) -> (x = y?=w63:bool)
  n63 = Equal?(x=1.0, y=w98) -> (x = y?=w64:bool)
  n64 = Equal?(x=1.0, y=w97) -> (x = y?=w65:bool)
  n65 = Equal?(x=1.0, y=w96) -> (x = y?=w66:bool)
  n66 = Equal?(x=1.0, y=w95) -> (x = y?=w88:bool)
  n67 = Index Array(array=w307) -> (element #1=w306:string, element #2=w305:string, element #3=w304:string, element #4=w303:string, element #5=w302:string, element #6=w301:string)  [unwired: 6 in]
  n68 = Select(t=TRUE, s=w65, f=FALSE) -> (s? t:f=w20:bool)
  n69 = Select(t=TRUE, s=w63, f=FALSE) -> (s? t:f=w18:bool)
  n70 = Select(t=TRUE, s=w64, f=FALSE) -> (s? t:f=w19:bool)
  n71 = Select(t=TRUE, s=w88, f=FALSE) -> (s? t:f=w22:bool)
  n72 = Select(t=TRUE, s=w60, f=FALSE) -> (s? t:f=w15:bool)
  n73 = Select(t=TRUE, s=w66, f=FALSE) -> (s? t:f=w21:bool)
  n74 = Unbundle By Name("main ref") -> ("Config Parameters.SAMPLES"=w331:refnum<vi>)
  n75 = Unbundle By Name("main ref") -> ("Config Parameters.Heave Loop Delay"=w219:refnum<vi>)
  n76 = Unbundle By Name("main ref") -> ("Config Parameters.Heave PID Speed"=w220:refnum<vi>)
  n77 = Unbundle By Name("main ref") -> ("Config Parameters.Surge Jog Speed"=w224:refnum<vi>)
  n78 = Unbundle By Name("main ref") -> ("Config Parameters.Heave Jog Speed"=w225:refnum<vi>)
  n79 = Unbundle By Name("main ref") -> ("About Screen.Humidity Port:"=w325:refnum<vi>)
  n80 = Unbundle By Name("main ref") -> ("About Screen.Temp Modbus:"=w320:refnum<vi>)
  n81 = Unbundle By Name("main ref") -> ("About Screen.Heave and Surge COM Port:"=w319:refnum<vi>)
  n82 = Unbundle By Name("main ref") -> ("About Screen.Sway COM Port:"=w315:refnum<vi>)
  n83 = Unbundle By Name("main ref") -> ("About Screen.Ramp Port:"=w314:refnum<vi>)
  n84 = Unbundle By Name("main ref") -> ("About Screen.ECR Port:"=w311:refnum<vi>)
  n85 = Unbundle By Name("main ref") -> ("Config Parameters.Sway PPR"=w392:refnum<vi>)
  n86 = Unbundle By Name("main ref") -> ("Config Parameters.Sway Pitch"=w387:refnum<vi>)
  n87 = Unbundle By Name("main ref") -> ("Config Parameters.Surge PPR"=w381:refnum<vi>)
  n88 = Unbundle By Name("main ref") -> ("Config Parameters.Surge Pitch"=w386:refnum<vi>)
  n89 = Unbundle By Name("main ref") -> ("Config Parameters.Heave PPR"=w380:refnum<vi>)
  n90 = Unbundle By Name("main ref") -> ("Config Parameters.Heave Pitch"=w376:refnum<vi>)
  n91 = Unbundle By Name("main ref") -> ("Config Parameters.Heave distance"=w370:refnum<vi>)
  n92 = Unbundle By Name("main ref") -> ("Config Parameters.Surge distance (mm)"=w374:refnum<vi>)
  n93 = Unbundle By Name("main ref") -> ("Config Parameters.Sway distance (mm)"=w368:refnum<vi>)
  n94 = Unbundle By Name("main ref") -> ("Config Parameters.DataSavingLoopDelay(ms)"=w365:refnum<vi>)
  n95 = Unbundle By Name("main ref") -> ("Config Parameters.Acoustic Emission:"=w362:refnum<vi>)
  n96 = Unbundle By Name("main ref") -> ("Config Parameters.RotHomeSurgeOffsetCounts"=w359:refnum<vi>)
  n97 = Unbundle By Name("main ref") -> ("Config Parameters.RotHomeSwayOffsetCounts"=w356:refnum<vi>)
  n98 = Unbundle By Name("main ref") -> ("Config Parameters.TracHomeSurgeOffsetCounts 20MM"=w353:refnum<vi>)
  n99 = Unbundle By Name("main ref") -> ("Config Parameters.TracHomeSwayOffsetCounts 20MM"=w350:refnum<vi>)
  n100 = Unbundle By Name("main ref") -> ("Config Parameters.TracHomeSurgeOffsetCounts 10MM"=w346:refnum<vi>)
  n101 = Unbundle By Name("main ref") -> ("Config Parameters.TracHomeSwayOffsetCounts 10MM"=w349:refnum<vi>)
  n102 = Unbundle By Name("main ref") -> ("Config Parameters.LRMHomeSurgeOffsetCounts"=w340:refnum<vi>)
  n103 = Unbundle By Name("main ref") -> ("Config Parameters.LRMHomeSwayOffsetCounts"=w337:refnum<vi>)
  n104 = Unbundle By Name("main ref") -> ("Config Parameters.Filter%"=w336:refnum<vi>)
  n105 = Unbundle By Name("main ref") -> ("Config Parameters.Filter% 2"=w332:refnum<vi>)
  n106 = Unbundle By Name("main ref") -> ("Config Parameters.LOAD TRIP  ENABLE"=w109:refnum<vi>)
  n107 = Unbundle By Name("main ref") -> ("Config Parameters.DEPTH TRIP VALUE"=w110:refnum<vi>)
  n108 = Unbundle By Name("main ref") -> ("Config Parameters.LOAD TRIP VALUE"=w114:refnum<vi>)
  n109 = Unbundle By Name("main ref") -> ("Config Parameters.DEPTH TRIP   ENABLE"=w115:refnum<vi>)
  n110 = Unbundle By Name("main ref") -> ("Config Parameters.CYCLIC FF TRIP VALUE"=w121:refnum<vi>)
  n111 = Unbundle By Name("main ref") -> ("Config Parameters.FF TRIP VALUE"=w122:refnum<vi>)
  n112 = Unbundle By Name("main ref") -> ("Config Parameters.CYCLIC CoF TRIP VALUE"=w127:refnum<vi>)
  n113 = Unbundle By Name("main ref") -> ("Config Parameters.CYCLIC FF TRIP  ENABLE"=w128:refnum<vi>)
  n114 = Unbundle By Name("main ref") -> ("Config Parameters.FF TRIP  ENABLE"=w136:refnum<vi>)
  n115 = Unbundle By Name("main ref") -> ("Config Parameters.COF TRIP  ENABLE"=w131:refnum<vi>)
  n116 = Unbundle By Name("main ref") -> ("Config Parameters.CYCLIC COF TRIP  ENABLE"=w104:refnum<vi>)
  n117 = Unbundle By Name("main ref") -> ("Config Parameters.COF TRIP VALUE"=w103:refnum<vi>)
  n118 = Unbundle By Name("main ref") -> ("Config Parameters.Sway Loop Delay"=w151:refnum<vi>)
  n119 = Unbundle By Name("main ref") -> ("Config Parameters.Sway PID Speed"=w147:refnum<vi>)
  n120 = Unbundle By Name("main ref") -> ("Config Parameters.Sway Jog Speed"=w146:refnum<vi>)
  n121 = property class="VISAName"(reference=w325, "Value"=w306) -> (reference out=w323:refnum<vi>, error out=w324:errorcluster)  [unwired: 1 in]
  n122 = property class="VISAName"(reference=w320, "Value"=w305) -> (reference out=w322:refnum<vi>, error out=w321:errorcluster)  [unwired: 1 in]
  n123 = Fract/Exp String To Number(string=w299) -> (number=w277:dbl)  [unwired: 3 in, 1 out]
  n124 = Fract/Exp String To Number(string=w298) -> (number=w276:dbl)  [unwired: 3 in, 1 out]
  n125 = Fract/Exp String To Number(string=w297) -> (number=w275:dbl)  [unwired: 3 in, 1 out]
  n126 = Fract/Exp String To Number(string=w296) -> (number=w274:dbl)  [unwired: 3 in, 1 out]
  n127 = Fract/Exp String To Number(string=w295) -> (number=w273:dbl)  [unwired: 3 in, 1 out]
  n128 = Fract/Exp String To Number(string=w294) -> (number=w272:dbl)  [unwired: 3 in, 1 out]
  n129 = Fract/Exp String To Number(string=w293) -> (number=w271:dbl)  [unwired: 3 in, 1 out]
  n130 = Fract/Exp String To Number(string=w292) -> (number=w270:dbl)  [unwired: 3 in, 1 out]
  n131 = Fract/Exp String To Number(string=w291) -> (number=w269:dbl)  [unwired: 3 in, 1 out]
  n132 = Fract/Exp String To Number(string=w290) -> (number=w268:dbl)  [unwired: 3 in, 1 out]
  n133 = Fract/Exp String To Number(string=w289) -> (number=w267:dbl)  [unwired: 3 in, 1 out]
  n134 = Fract/Exp String To Number(string=w288) -> (number=w266:dbl)  [unwired: 3 in, 1 out]
  n135 = Fract/Exp String To Number(string=w287) -> (number=w265:dbl)  [unwired: 3 in, 1 out]
  n136 = Fract/Exp String To Number(string=w286) -> (number=w264:dbl)  [unwired: 3 in, 1 out]
  n137 = Fract/Exp String To Number(string=w285) -> (number=w263:dbl)  [unwired: 3 in, 1 out]
  n138 = Fract/Exp String To Number(string=w284) -> (number=w262:dbl)  [unwired: 3 in, 1 out]
  n139 = Fract/Exp String To Number(string=w283) -> (number=w261:dbl)  [unwired: 3 in, 1 out]
  n140 = Fract/Exp String To Number(string=w282) -> (number=w260:dbl)  [unwired: 3 in, 1 out]
  n141 = Fract/Exp String To Number(string=w281) -> (number=w259:dbl)  [unwired: 3 in, 1 out]
  n142 = Fract/Exp String To Number(string=w280) -> (number=w258:dbl)  [unwired: 3 in, 1 out]
  n143 = Fract/Exp String To Number(string=w279) -> (number=w257:dbl)  [unwired: 3 in, 1 out]
  n144 = Fract/Exp String To Number(string=w278) -> (number=w256:dbl)  [unwired: 3 in, 1 out]
  n145 = Fract/Exp String To Number(string=w216) -> (number=w229:dbl)  [unwired: 3 in, 1 out]
  n146 = Fract/Exp String To Number(string=w215) -> (number=w230:dbl)  [unwired: 3 in, 1 out]
  n147 = Fract/Exp String To Number(string=w214) -> (number=w231:dbl)  [unwired: 3 in, 1 out]
  n148 = Fract/Exp String To Number(string=w213) -> (number=w232:dbl)  [unwired: 3 in, 1 out]
  n149 = Fract/Exp String To Number(string=w23) -> (number=w10:dbl)  [unwired: 3 in, 1 out]
  n150 = Fract/Exp String To Number(string=w87) -> (number=w14:dbl)  [unwired: 3 in, 1 out]
  n151 = Fract/Exp String To Number(string=w84) -> (number=w16:dbl)  [unwired: 3 in, 1 out]
  n152 = Fract/Exp String To Number(string=w86) -> (number=w6:dbl)  [unwired: 3 in, 1 out]
  n153 = Fract/Exp String To Number(string=w82) -> (number=w17:dbl)  [unwired: 3 in, 1 out]
  n154 = Fract/Exp String To Number(string=w139) -> (number=w142:dbl)  [unwired: 3 in, 1 out]
  n155 = Fract/Exp String To Number(string=w138) -> (number=w141:dbl)  [unwired: 3 in, 1 out]
  n156 = Fract/Exp String To Number(string=w137) -> (number=w140:dbl)  [unwired: 3 in, 1 out]
  n157 = property class="VISAName"(reference=w319, "Value"=w304) -> (reference out=w317:refnum<vi>, error out=w318:errorcluster)  [unwired: 1 in]
  n158 = property class="VISAName"(reference=w315, "Value"=w303) -> (reference out=w310:refnum<vi>, error out=w316:errorcluster)  [unwired: 1 in]
  n159 = property class="VISAName"(reference=w314, "Value"=w302) -> (reference out=w309:refnum<vi>, error out=w313:errorcluster)  [unwired: 1 in]
  n160 = property class="VISAName"(reference=w311, "Value"=w301) -> (reference out=w308:refnum<vi>, error out=w312:errorcluster)  [unwired: 1 in]
  n161 = Fract/Exp String To Number(string=w83) -> (number=w1:dbl)  [unwired: 3 in, 1 out]
  n162 = property class="DigNum (strict)"(reference=w340, "Value"=w260) -> (reference out=w341:refnum<vi>, error out=w339:errorcluster)  [unwired: 1 in]
  n163 = property class="DigNum (strict)"(reference=w337, "Value"=w259) -> (reference out=w342:refnum<vi>, error out=w338:errorcluster)  [unwired: 1 in]
  n164 = property class="DigNum (strict)"(reference=w336, "Value"=w258) -> (reference out=w334:refnum<vi>, error out=w335:errorcluster)  [unwired: 1 in]
  n165 = property class="DigNum (strict)"(reference=w331, "Value"=w256) -> (reference out=w329:refnum<vi>, error out=w330:errorcluster)  [unwired: 1 in]
  n166 = property class="DigNum (strict)"(reference=w219, "Value"=w229) -> (reference out=w217:refnum<vi>, error out=w218:errorcluster)  [unwired: 1 in]
  n167 = property class="DigNum (strict)"(reference=w332, "Value"=w257) -> (reference out=w328:refnum<vi>, error out=w333:errorcluster)  [unwired: 1 in]
  n168 = property class="DigNum (strict)"(reference=w220, "Value"=w230) -> (reference out=w222:refnum<vi>, error out=w221:errorcluster)  [unwired: 1 in]
  n169 = property class="DigNum (strict)"(reference=w225, "Value"=w232) -> (reference out=w227:refnum<vi>, error out=w226:errorcluster)  [unwired: 1 in]
  n170 = property class="DigNum (strict)"(reference=w356, "Value"=w265) -> (reference out=w355:refnum<vi>, error out=w357:errorcluster)  [unwired: 1 in]
  n171 = property class="DigNum (strict)"(reference=w346, "Value"=w262) -> (reference out=w344:refnum<vi>, error out=w347:errorcluster)  [unwired: 1 in]
  n172 = property class="DigNum (strict)"(reference=w349, "Value"=w261) -> (reference out=w343:refnum<vi>, error out=w348:errorcluster)  [unwired: 1 in]
  n173 = property class="DigNum (strict)"(reference=w224, "Value"=w231) -> (reference out=w228:refnum<vi>, error out=w223:errorcluster)  [unwired: 1 in]
  n174 = property class="DigNum (strict)"(reference=w392, "Value"=w277) -> (reference out=w390:refnum<vi>, error out=w391:errorcluster)  [unwired: 1 in]
  n175 = property class="DigNum (strict)"(reference=w370, "Value"=w271) -> (reference out=w327:refnum<vi>, error out=w371:errorcluster)  [unwired: 1 in]
  n176 = property class="DigNum (strict)"(reference=w353, "Value"=w264) -> (reference out=w354:refnum<vi>, error out=w352:errorcluster)  [unwired: 1 in]
  n177 = property class="DigNum (strict)"(reference=w350, "Value"=w263) -> (reference out=w345:refnum<vi>, error out=w351:errorcluster)  [unwired: 1 in]
  n178 = property class="DigNum (strict)"(reference=w387, "Value"=w276) -> (reference out=w389:refnum<vi>, error out=w388:errorcluster)  [unwired: 1 in]
  n179 = property class="DigNum (strict)"(reference=w381, "Value"=w275) -> (reference out=w383:refnum<vi>, error out=w382:errorcluster)  [unwired: 1 in]
  n180 = property class="DigNum (strict)"(reference=w380, "Value"=w273) -> (reference out=w375:refnum<vi>, error out=w379:errorcluster)  [unwired: 1 in]
  n181 = property class="DigNum (strict)"(reference=w374, "Value"=w270) -> (reference out=w372:refnum<vi>, error out=w373:errorcluster)  [unwired: 1 in]
  n182 = property class="DigNum (strict)"(reference=w368, "Value"=w269) -> (reference out=w367:refnum<vi>, error out=w369:errorcluster)  [unwired: 1 in]
  n183 = property class="DigNum (strict)"(reference=w365, "Value"=w268) -> (reference out=w366:refnum<vi>, error out=w364:errorcluster)  [unwired: 1 in]
  n184 = property class="DigNum (strict)"(reference=w362, "Value"=w267) -> (reference out=w361:refnum<vi>, error out=w363:errorcluster)  [unwired: 1 in]
  n185 = property class="DigNum (strict)"(reference=w359, "Value"=w266) -> (reference out=w360:refnum<vi>, error out=w358:errorcluster)  [unwired: 1 in]
  n186 = property class="DigNum (strict)"(reference=w386, "Value"=w274) -> (reference out=w384:refnum<vi>, error out=w385:errorcluster)  [unwired: 1 in]
  n187 = property class="DigNum (strict)"(reference=w376, "Value"=w272) -> (reference out=w378:refnum<vi>, error out=w377:errorcluster)  [unwired: 1 in]
  n188 = property class="DigNum (strict)"(reference=w151, "Value"=w142) -> (reference out=w149:refnum<vi>, error out=w150:errorcluster)  [unwired: 1 in]
  n189 = property class="DigNum (strict)"(reference=w146, "Value"=w140) -> (reference out=w144:refnum<vi>, error out=w145:errorcluster)  [unwired: 1 in]
  n190 = property class="DigNum (strict)"(reference=w110, "Value"=w14) -> (reference out=w112:refnum<vi>, error out=w111:errorcluster)  [unwired: 1 in]
  n191 = property class="DigNum (strict)"(reference=w121, "Value"=w16) -> (reference out=w119:refnum<vi>, error out=w120:errorcluster)  [unwired: 1 in]
  n192 = property class="DigNum (strict)"(reference=w122, "Value"=w1) -> (reference out=w124:refnum<vi>, error out=w123:errorcluster)  [unwired: 1 in]
  n193 = property class="DigNum (strict)"(reference=w127, "Value"=w17) -> (reference out=w125:refnum<vi>, error out=w126:errorcluster)  [unwired: 1 in]
  n194 = property class="DigNum (strict)"(reference=w147, "Value"=w141) -> (reference out=w143:refnum<vi>, error out=w148:errorcluster)  [unwired: 1 in]
  n195 = property class="DigNum (strict)"(reference=w114, "Value"=w6) -> (reference out=w118:refnum<vi>, error out=w113:errorcluster)  [unwired: 1 in]
  n196 = property class="Bool (strict)"(reference=w104, "Value"=w22) -> (reference out=w106:refnum<vi>, error out=w105:errorcluster)  [unwired: 1 in]
  n197 = property class="DigNum (strict)"(reference=w103, "Value"=w10) -> (reference out=w101:refnum<vi>, error out=w102:errorcluster)  [unwired: 1 in]
  n198 = property class="Bool (strict)"(reference=w115, "Value"=w15) -> (reference out=w117:refnum<vi>, error out=w116:errorcluster)  [unwired: 1 in]
  n199 = property class="Bool (strict)"(reference=w128, "Value"=w18) -> (reference out=w130:refnum<vi>, error out=w129:errorcluster)  [unwired: 1 in]
  n200 = property class="Bool (strict)"(reference=w136, "Value"=w19) -> (reference out=w134:refnum<vi>, error out=w135:errorcluster)  [unwired: 1 in]
  n201 = property class="Bool (strict)"(reference=w131, "Value"=w20) -> (reference out=w133:refnum<vi>, error out=w132:errorcluster)  [unwired: 1 in]
  n202 = property class="Bool (strict)"(reference=w109, "Value"=w21) -> (reference out=w107:refnum<vi>, error out=w108:errorcluster)  [unwired: 1 in]
  n203 = Close Reference(reference=w323, error in (no error)=w324) -> ()  [unwired: 1 out]
  n204 = Close Reference(reference=w322, error in (no error)=w321) -> ()  [unwired: 1 out]
  n205 = Close Reference(reference=w317, error in (no error)=w318) -> ()  [unwired: 1 out]
  n206 = Close Reference(reference=w310, error in (no error)=w316) -> ()  [unwired: 1 out]
  n207 = Close Reference(reference=w309, error in (no error)=w313) -> ()  [unwired: 1 out]
  n208 = Close Reference(reference=w308, error in (no error)=w312) -> ()  [unwired: 1 out]
  n209 = Close Reference(reference=w341, error in (no error)=w339) -> ()  [unwired: 1 out]
  n210 = Close Reference(reference=w342, error in (no error)=w338) -> ()  [unwired: 1 out]
  n211 = Close Reference(reference=w334, error in (no error)=w335) -> ()  [unwired: 1 out]
  n212 = Close Reference(reference=w329, error in (no error)=w330) -> ()  [unwired: 1 out]
  n213 = Close Reference(reference=w217, error in (no error)=w218) -> ()  [unwired: 1 out]
  n214 = Close Reference(reference=w328, error in (no error)=w333) -> ()  [unwired: 1 out]
  n215 = Close Reference(reference=w222, error in (no error)=w221) -> ()  [unwired: 1 out]
  n216 = Close Reference(reference=w227, error in (no error)=w226) -> ()  [unwired: 1 out]
  n217 = Close Reference(reference=w355, error in (no error)=w357) -> ()  [unwired: 1 out]
  n218 = Close Reference(reference=w344, error in (no error)=w347) -> ()  [unwired: 1 out]
  n219 = Close Reference(reference=w343, error in (no error)=w348) -> ()  [unwired: 1 out]
  n220 = Close Reference(reference=w228, error in (no error)=w223) -> ()  [unwired: 1 out]
  n221 = Close Reference(reference=w390, error in (no error)=w391) -> ()  [unwired: 1 out]
  n222 = Close Reference(reference=w327, error in (no error)=w371) -> ()  [unwired: 1 out]
  n223 = Close Reference(reference=w354, error in (no error)=w352) -> ()  [unwired: 1 out]
  n224 = Close Reference(reference=w345, error in (no error)=w351) -> ()  [unwired: 1 out]
  n225 = Close Reference(reference=w389, error in (no error)=w388) -> ()  [unwired: 1 out]
  n226 = Close Reference(reference=w383, error in (no error)=w382) -> ()  [unwired: 1 out]
  n227 = Close Reference(reference=w375, error in (no error)=w379) -> ()  [unwired: 1 out]
  n228 = Close Reference(reference=w372, error in (no error)=w373) -> ()  [unwired: 1 out]
  n229 = Close Reference(reference=w367, error in (no error)=w369) -> ()  [unwired: 1 out]
  n230 = Close Reference(reference=w366, error in (no error)=w364) -> ()  [unwired: 1 out]
  n231 = Close Reference(reference=w361, error in (no error)=w363) -> ()  [unwired: 1 out]
  n232 = Close Reference(reference=w360, error in (no error)=w358) -> ()  [unwired: 1 out]
  n233 = Close Reference(reference=w384, error in (no error)=w385) -> ()  [unwired: 1 out]
  n234 = Close Reference(reference=w378, error in (no error)=w377) -> ()  [unwired: 1 out]
  n235 = Close Reference(reference=w106, error in (no error)=w105) -> ()  [unwired: 1 out]
  n236 = Close Reference(reference=w149, error in (no error)=w150) -> ()  [unwired: 1 out]
  n237 = Close Reference(reference=w144, error in (no error)=w145) -> ()  [unwired: 1 out]
  n238 = Close Reference(reference=w112, error in (no error)=w111) -> ()  [unwired: 1 out]
  n239 = Close Reference(reference=w117, error in (no error)=w116) -> ()  [unwired: 1 out]
  n240 = Close Reference(reference=w119, error in (no error)=w120) -> ()  [unwired: 1 out]
  n241 = Close Reference(reference=w124, error in (no error)=w123) -> ()  [unwired: 1 out]
  n242 = Close Reference(reference=w125, error in (no error)=w126) -> ()  [unwired: 1 out]
  n243 = Close Reference(reference=w130, error in (no error)=w129) -> ()  [unwired: 1 out]
  n244 = Close Reference(reference=w134, error in (no error)=w135) -> ()  [unwired: 1 out]
  n245 = Close Reference(reference=w133, error in (no error)=w132) -> ()  [unwired: 1 out]
  n246 = Close Reference(reference=w107, error in (no error)=w108) -> ()  [unwired: 1 out]
  n247 = Close Reference(reference=w143, error in (no error)=w148) -> ()  [unwired: 1 out]
  n248 = Close Reference(reference=w118, error in (no error)=w113) -> ()  [unwired: 1 out]
  n249 = Close Reference(reference=w101, error in (no error)=w102) -> ()  [unwired: 1 out]
  n250 = for {
    tunnel: "NEW PID PARAMETERS" ("WRITE /READ SECTION") -> [w467]
    tunnel: [w466] -> w210
    tunnel: string[] ["PID DELAY (sec)", "Kp", "Ki", "Kd", "Deaadband", "pct_scale", "Init_step", "i_limit", "Max Step Limit", "Min_pos_limit", "Max_pos_limit", "Fine_tune_zone"] -> [w463] mode=indexing
    tunnel: [w462] -> w182 mode=indexing
    tunnel: w211 -> [w461]
    n251 = call "CONFIG FILE MAIN Unitest.vi"("WRITE /READ SECTION"=w467, "READ KEY"=w463, "error in"=w461, "PARAMETER/CONFIG"=TRUE, "Config Enum"=Config_file__FGV_Unitest_enum."READ") -> ("READ VALUE"=w462:string, "error out"=w466:errorcluster)  [unwired: 13 in]
  }
  n252 = Unbundle By Name("main ref") -> ("Loading.Enter the CoF Trip"=w13:refnum<vi>)
  n253 = Unbundle By Name("main ref") -> ("Main Screen.Load Disable Trip"=w51:refnum<vi>)
  n254 = Unbundle By Name("main ref") -> ("Main Screen.FF Disable Trip"=w24:refnum<vi>)
  n255 = Unbundle By Name("main ref") -> ("Main Screen.COF Disable Trip"=w29:refnum<vi>)
  n256 = Unbundle By Name("main ref") -> ("Main Screen.Cyclic FF Disable Trip"=w32:refnum<vi>)
  n257 = Unbundle By Name("main ref") -> ("Main Screen.cyclic COF Disable Trip"=w56:refnum<vi>)
  n258 = Unbundle By Name("main ref") -> ("Main Screen.FF TRIP"=w38:refnum<vi>)
  n259 = Unbundle By Name("main ref") -> ("Main Screen.COF TRIP"=w57:refnum<vi>)
  n260 = Unbundle By Name("main ref") -> ("Main Screen.Depth Trip"=w50:refnum<vi>)
  n261 = Unbundle By Name("main ref") -> ("Main Screen.Depth Trip 2"=w45:refnum<vi>)
  n262 = Unbundle By Name("main ref") -> ("Main Screen.Cyclic FF TRIP"=w39:refnum<vi>)
  n263 = Unbundle By Name("main ref") -> ("Main Screen.cyclic COF TRIP"=w33:refnum<vi>)
  n264 = Unbundle By Name("main ref") -> ("Main Screen.NL Trip 2"=w46:refnum<vi>)
  n265 = Unbundle By Name("main ref") -> ("New PID LOGIC.PID SDelay"=w206:refnum<vi>)
  n266 = Unbundle By Name("main ref") -> ("New PID LOGIC.Kp"=w205:refnum<vi>)
  n267 = Unbundle By Name("main ref") -> ("New PID LOGIC.Ki"=w200:refnum<vi>)
  n268 = Unbundle By Name("main ref") -> ("New PID LOGIC.Kd"=w199:refnum<vi>)
  n269 = Unbundle By Name("main ref") -> ("New PID LOGIC.Deadband"=w195:refnum<vi>)
  n270 = Unbundle By Name("main ref") -> ("New PID LOGIC.pct_scale"=w194:refnum<vi>)
  n271 = Unbundle By Name("main ref") -> ("New PID LOGIC.Init Step"=w191:refnum<vi>)
  n272 = Unbundle By Name("main ref") -> ("New PID LOGIC.i_limit"=w190:refnum<vi>)
  n273 = Unbundle By Name("main ref") -> ("New PID LOGIC.Max Step Linit"=w187:refnum<vi>)
  n274 = Unbundle By Name("main ref") -> ("New PID LOGIC.Max_pos_limit"=w185:refnum<vi>)
  n275 = Unbundle By Name("main ref") -> ("New PID LOGIC.Min_pos_limit"=w184:refnum<vi>)
  n276 = Index Array(array=w182) -> (element #1=w181:string, element #2=w180:string, element #3=w177:string, element #4=w176:string, element #5=w175:string, element #6=w174:string, element #7=w169:string, element #8=w168:string, element #9=w167:string, element #10=w166:string, element #11=w165:string)  [unwired: 11 in]
  n277 = property class="DigNum (strict)"(reference=w13, "Value"=w10) -> (reference out=w11:refnum<vi>, error out=w12:errorcluster)  [unwired: 1 in]
  n278 = property class="DigNum (strict)"(reference=w50, "Value"=w14) -> (reference out=w48:refnum<vi>, error out=w49:errorcluster)  [unwired: 1 in]
  n279 = property class="DigNum (strict)"(reference=w39, "Value"=w16) -> (reference out=w41:refnum<vi>, error out=w40:errorcluster)  [unwired: 1 in]
  n280 = property class="DigNum (strict)"(reference=w38, "Value"=w1) -> (reference out=w36:refnum<vi>, error out=w37:errorcluster)  [unwired: 1 in]
  n281 = property class="DigNum (strict)"(reference=w33, "Value"=w17) -> (reference out=w35:refnum<vi>, error out=w34:errorcluster)  [unwired: 1 in]
  n282 = property class="DigNum (strict)"(reference=w46, "Value"=w6) -> (reference out=w42:refnum<vi>, error out=w47:errorcluster)  [unwired: 1 in]
  n283 = property class="Bool (strict)"(reference=w56, "Value"=w22) -> (reference out=w54:refnum<vi>, error out=w55:errorcluster)  [unwired: 1 in]
  n284 = property class="DigNum (strict)"(reference=w57, "Value"=w10) -> (reference out=w59:refnum<vi>, error out=w58:errorcluster)  [unwired: 1 in]
  n285 = property class="Bool (strict)"(reference=w45, "Value"=w15) -> (reference out=w43:refnum<vi>, error out=w44:errorcluster)  [unwired: 1 in]
  n286 = property class="Bool (strict)"(reference=w32, "Value"=w18) -> (reference out=w30:refnum<vi>, error out=w31:errorcluster)  [unwired: 1 in]
  n287 = property class="Bool (strict)"(reference=w24, "Value"=w19) -> (reference out=w26:refnum<vi>, error out=w25:errorcluster)  [unwired: 1 in]
  n288 = property class="Bool (strict)"(reference=w29, "Value"=w20) -> (reference out=w27:refnum<vi>, error out=w28:errorcluster)  [unwired: 1 in]
  n289 = property class="Bool (strict)"(reference=w51, "Value"=w21) -> (reference out=w53:refnum<vi>, error out=w52:errorcluster)  [unwired: 1 in]
  n290 = call "CONFIG FILE MAIN Unitest.vi"("error in"=w210, "Config Enum"=Config_file__FGV_Unitest_enum."CLOSE") -> ("error out"=→"error out":errorcluster)  [unwired: 16 in, 1 out]
  n291 = Unbundle By Name("main ref") -> ("Loading.Enter the Normal load Trip"=w9:refnum<vi>)
  n292 = Fract/Exp String To Number(string=w181) -> (number=w179:dbl)  [unwired: 3 in, 1 out]
  n293 = Fract/Exp String To Number(string=w180) -> (number=w178:dbl)  [unwired: 3 in, 1 out]
  n294 = Fract/Exp String To Number(string=w177) -> (number=w173:dbl)  [unwired: 3 in, 1 out]
  n295 = Close Reference(reference=w11, error in (no error)=w12) -> ()  [unwired: 1 out]
  n296 = Fract/Exp String To Number(string=w176) -> (number=w172:dbl)  [unwired: 3 in, 1 out]
  n297 = Fract/Exp String To Number(string=w175) -> (number=w171:dbl)  [unwired: 3 in, 1 out]
  n298 = Fract/Exp String To Number(string=w174) -> (number=w170:dbl)  [unwired: 3 in, 1 out]
  n299 = Fract/Exp String To Number(string=w169) -> (number=w164:dbl)  [unwired: 3 in, 1 out]
  n300 = Fract/Exp String To Number(string=w168) -> (number=w163:dbl)  [unwired: 3 in, 1 out]
  n301 = Fract/Exp String To Number(string=w167) -> (number=w162:dbl)  [unwired: 3 in, 1 out]
  n302 = Fract/Exp String To Number(string=w166) -> (number=w161:dbl)  [unwired: 3 in, 1 out]
  n303 = Fract/Exp String To Number(string=w165) -> (number=w160:dbl)  [unwired: 3 in, 1 out]
  n304 = Close Reference(reference=w54, error in (no error)=w55) -> ()  [unwired: 1 out]
  n305 = Unbundle By Name("main ref") -> ("Loading.Enter the Friction Force Trip"=w5:refnum<vi>)
  n306 = Close Reference(reference=w48, error in (no error)=w49) -> ()  [unwired: 1 out]
  n307 = Close Reference(reference=w43, error in (no error)=w44) -> ()  [unwired: 1 out]
  n308 = Close Reference(reference=w41, error in (no error)=w40) -> ()  [unwired: 1 out]
  n309 = Close Reference(reference=w36, error in (no error)=w37) -> ()  [unwired: 1 out]
  n310 = Close Reference(reference=w35, error in (no error)=w34) -> ()  [unwired: 1 out]
  n311 = Close Reference(reference=w30, error in (no error)=w31) -> ()  [unwired: 1 out]
  n312 = Close Reference(reference=w26, error in (no error)=w25) -> ()  [unwired: 1 out]
  n313 = Close Reference(reference=w27, error in (no error)=w28) -> ()  [unwired: 1 out]
  n314 = Close Reference(reference=w53, error in (no error)=w52) -> ()  [unwired: 1 out]
  n315 = Close Reference(reference=w42, error in (no error)=w47) -> ()  [unwired: 1 out]
  n316 = Close Reference(reference=w59, error in (no error)=w58) -> ()  [unwired: 1 out]
  n317 = property class="DigNum (strict)"(reference=w206, "Value"=w179) -> (reference out=w208:refnum<vi>, error out=w207:errorcluster)  [unwired: 1 in]
  n318 = property class="DigNum (strict)"(reference=w205, "Value"=w178) -> (reference out=w203:refnum<vi>, error out=w204:errorcluster)  [unwired: 1 in]
  n319 = property class="DigNum (strict)"(reference=w200, "Value"=w173) -> (reference out=w202:refnum<vi>, error out=w201:errorcluster)  [unwired: 1 in]
  n320 = property class="DigNum (strict)"(reference=w199, "Value"=w172) -> (reference out=w197:refnum<vi>, error out=w198:errorcluster)  [unwired: 1 in]
  n321 = property class="DigNum (strict)"(reference=w195, "Value"=w171) -> (reference out=w158:refnum<vi>, error out=w196:errorcluster)  [unwired: 1 in]
  n322 = property class="DigNum (strict)"(reference=w194, "Value"=w170) -> (reference out=w159:refnum<vi>, error out=w193:errorcluster)  [unwired: 1 in]
  n323 = property class="DigNum (strict)"(reference=w191, "Value"=w164) -> (reference out=w157:refnum<vi>, error out=w192:errorcluster)  [unwired: 1 in]
  n324 = property class="DigNum (strict)"(reference=w190, "Value"=w163) -> (reference out=w156:refnum<vi>, error out=w189:errorcluster)  [unwired: 1 in]
  n325 = property class="DigNum (strict)"(reference=w187, "Value"=w162) -> (reference out=w155:refnum<vi>, error out=w188:errorcluster)  [unwired: 1 in]
  n326 = property class="DigNum (strict)"(reference=w185, "Value"=w161) -> (reference out=w154:refnum<vi>, error out=w186:errorcluster)  [unwired: 1 in]
  n327 = property class="DigNum (strict)"(reference=w184, "Value"=w160) -> (reference out=w153:refnum<vi>, error out=w183:errorcluster)  [unwired: 1 in]
  n328 = property class="DigNum (strict)"(reference=w9, "Value"=w6) -> (reference out=w7:refnum<vi>, error out=w8:errorcluster)  [unwired: 1 in]
  n329 = property class="DigNum (strict)"(reference=w5, "Value"=w1) -> (reference out=w3:refnum<vi>, error out=w4:errorcluster)  [unwired: 1 in]
  n330 = Close Reference(reference=w208, error in (no error)=w207) -> ()  [unwired: 1 out]
  n331 = Close Reference(reference=w203, error in (no error)=w204) -> ()  [unwired: 1 out]
  n332 = Close Reference(reference=w202, error in (no error)=w201) -> ()  [unwired: 1 out]
  n333 = Close Reference(reference=w197, error in (no error)=w198) -> ()  [unwired: 1 out]
  n334 = Close Reference(reference=w158, error in (no error)=w196) -> ()  [unwired: 1 out]
  n335 = Close Reference(reference=w159, error in (no error)=w193) -> ()  [unwired: 1 out]
  n336 = Close Reference(reference=w157, error in (no error)=w192) -> ()  [unwired: 1 out]
  n337 = Close Reference(reference=w156, error in (no error)=w189) -> ()  [unwired: 1 out]
  n338 = Close Reference(reference=w155, error in (no error)=w188) -> ()  [unwired: 1 out]
  n339 = Close Reference(reference=w154, error in (no error)=w186) -> ()  [unwired: 1 out]
  n340 = Close Reference(reference=w153, error in (no error)=w183) -> ()  [unwired: 1 out]
  n341 = Close Reference(reference=w7, error in (no error)=w8) -> ()  [unwired: 1 out]
  n342 = Close Reference(reference=w3, error in (no error)=w4) -> ()  [unwired: 1 out]
